vi "OCR Example.vi"() -> ()   [LabVIEW 2015]
doc: "This VI demonstrates how OCR could be used in an unstructured environment. Given the shape of surface that the text is printed on, LabVIEW can perform a perspective distortion correction to allow the OCR to better translate the text."
uses:
  <vilib>/userdefined/High Color/IMAQdx.ctl
  <vilib>/vision/driver/NI_Vision_Acquisition_Software.lvlib
  <resource>/objmgr/imaqdx.rc
  <vilib>/vision/NI_Vision_Development_Module.lvlib
panel:
  in  "stop":bool
  in  "Error in (no error)":errorcluster
  in  "Video Source":enum32{"File", "Live"}(radio)
  out "Camera Tab Control":enum32{"Pre-Loaded Video", "Live Camera"}(tab)
  in  "Frame Number":u32(slide) max=8 scale=0.0..8.0
  in  "Live Camera":T1="Select camera"
  in  "Video modes":u16(ring) items=["160x120 MJPG 30.00fps", "160x120 YUY2 30.00fps", "176x144 MJPG 30.00fps", "176x144 YUY2 30.00fps", "320x176 MJPG 30.00fps", "320x176 YUY2 30.00fps", "320x240 MJPG 30.00fps", "320x240 YUY2 30.00fps", "352x288 MJPG 30.00fps", "352x288 YUY2 30.00fps", "432x240 MJPG 30.00fps", "432x240 YUY2 30.00fps", "544x288 MJPG 30.00fps", "544x288 YUY2 30.00fps", "640x360 MJPG 30.00fps", "640x360 YUY2 30.00fps", "640x480 MJPG 30.00fps", "640x480 YUY2 30.00fps", "800x480 MJPG 30.00fps", "1024x768 MJPG 30.00fps"]
  in  "Start":bool
  in  "Tab Control":enum32{"Thresholding", "Corrected Feed"}(tab)=enum."Corrected Feed"
  out "Thresholded Image":T2(plugin-control)
  in  "Red or Hue":cluster{"Min":i32, "Max":i32}(slide)={"Min"=217, "Max"=15} scale=0.0..255.0
  in  "Green or Saturation":cluster{"Min":i32, "Max":i32}(slide)={"Min"=49, "Max"=165} scale=0.0..255.0
  in  "Blue or Luminance":cluster{"Min":i32, "Max":i32}(slide)={"Min"=65, "Max"=183} scale=0.0..255.0
  out "Corrected Feed":T2(plugin-control)
  in  "Relative Border Thickness":dbl(slide)=0.1274336283185841 scale=0.0..0.4 scale format="%.2g"
  out "OCR String":string
  out "Loop Time":i64
  in  "Apply correction":bool
  out "Original Feed":T2(plugin-control)
  # "This VI demonstrates how OCR could be used in an unstructured environment.\n  \n1. Select the video source before running the VI.\n2. Go through each frame without Apply correction toggled and notice when \nthe text is correctly identified.  \n3. Switch the image correction on.  Notice the change in Loop Time.\n\nThe video source must be live if using this example on an RT target.\nSee OCR Readme.html for more help and information."
  # "Use these sliders to adjust what color the \nVI identifies as the rectangle surrounding \nthe text."
  # "If using a Live video source, adjust the \nRelative Border Thickness so the green ROI\nlies completely within the red rectangle."
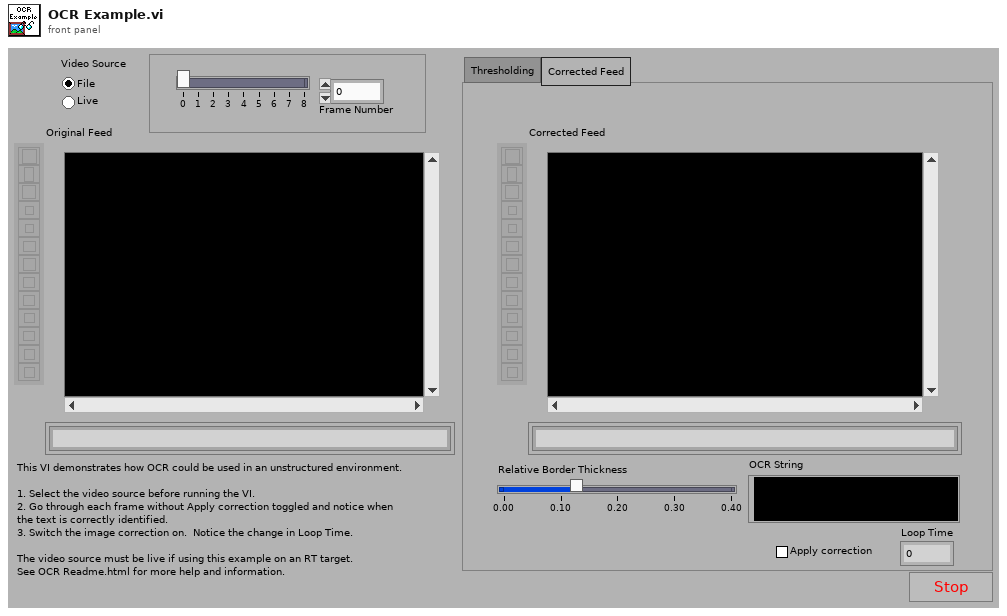
[diagram p1: front panel]
types:
  T1 = typedef "IMAQdx.ctl" = refnum<k21>
  T2 = typedef "IMAQ Image.ctl" = refnum<image>
  T3 = typedef "AviRefnum.ctl" = refnum<k1>
  T4 = typedef "IMAQ OCR Session.ctl" = refnum<k1>
  T5 = typedef "Image Type" = u32
  T6 = typedef "ROI Descriptor" = cluster{"Global Rectangle":i32[], "Contours":cluster{"ID":enum32{"External", "Internal"}, "Type":u32, "Coordinates":i32[]}[]}
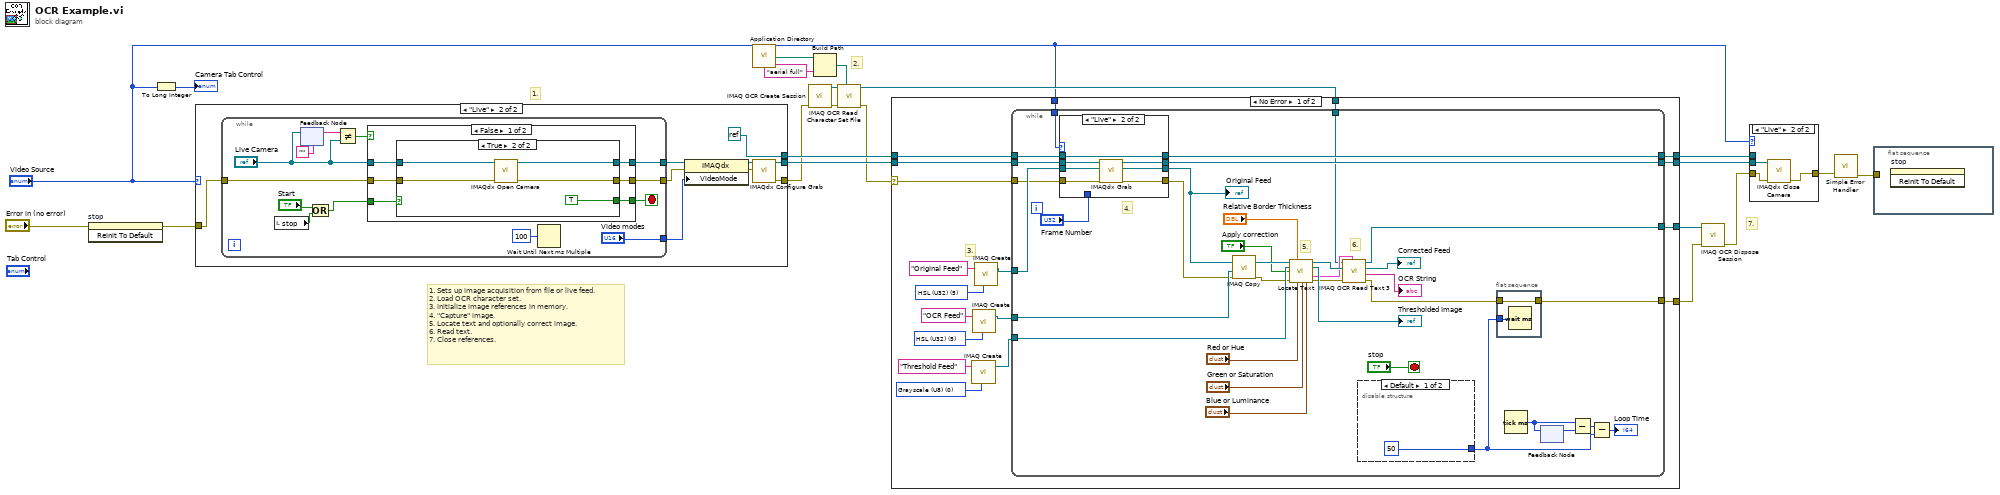
[diagram p0: block diagram]
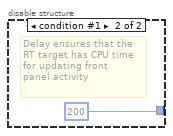
[diagram p2: hidden frame]
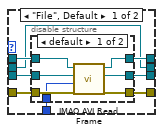
[diagram p3: hidden frame]
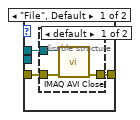
[diagram p6: hidden frame]
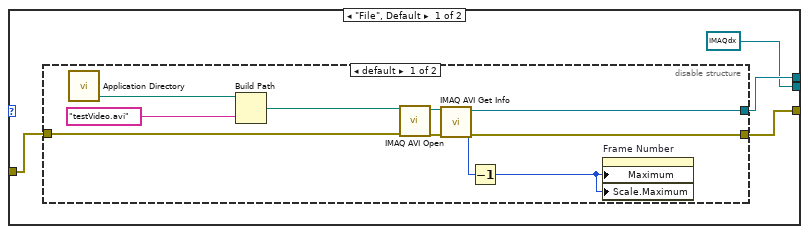
[diagram p8: hidden frame]
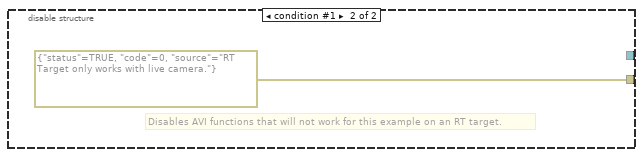
[diagram p9: hidden frame]
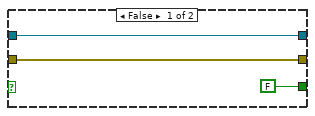
[diagram p10: hidden frame]
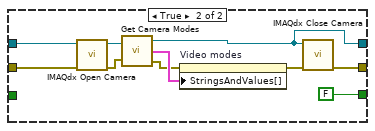
[diagram p11: hidden frame]
diagram:
  # "7."
  # "2."
  # "1."
  # "1. Sets up image acquisition from file or live feed.\n2. Load OCR character set.\n3. Initialize image references in memory.\n4. \"Capture\" image.\n5. Locate text and optionally correct image.\n6. Read text.\n7. Close references."
  n1 = invoke on="stop" class="Bool (strict)" method="Reinit To Default"(error in="Error in (no error)") -> (error out=w2:errorcluster)  [unwired: 2 in, 2 out]
  n2 = To Long Integer(number="Video Source") -> (32bit integer=→"Camera Tab Control":i32)
  n3 = case shown="\"Live\"" "Video Source" {
    tunnel: [T1 refnum ("Session Out") w45] -> w21
    tunnel: [w24 w42] -> w7
    tunnel: [w25 refnum<k0> refnum] -> w19
    tunnel: w2 -> [w23 w38]
    frame "File", Default {
      n4 = disable-structure shown="default" {
        disable-tunnel: [w34 _] -> w25
        disable-tunnel: [w33 errorcluster {"status"=TRUE, "code"=0, "source"="RT Target only works with live camera."} ("error out")] -> w24
        disable-tunnel: w23 -> [w26 _]
        frame condition #0 (active) {
          n5 = call <vilib>:"Application Directory.vi"() -> ("Application Directory"=w29:path)
          n6 = Build Path(base path=w29, name or relative path="testVideo.avi") -> (appended path=w27:path)
          n7 = call "IMAQ AVI Open"("error in (no error)"=w26, "AVI Path"=w27) -> ("error out"=w32:errorcluster, "Avi Refnum"=w35:T3)  [unwired: 8 in]
          n8 = call "IMAQ AVI Get Info"("error in (no error)"=w32, "Avi Refnum"=w35) -> ("error out"=w33:errorcluster, "Number of Frames"=w31:u32, "Avi Refnum (duplicate)"=w34:T3)  [unwired: 5 in, 2 out]
          n9 = Decrement(x=w31) -> (x-1=w30:u32)
          n10 = property on="Frame Number" class="Slide (strict)"("Maximum"=w30, "Scale.Maximum"=w30) -> ()  [unwired: 2 in, 2 out]
        }
        frame condition #1 {
          # "Disables AVI functions that will not work for this example on an RT target."
        }
      }
    }
    frame "Live" {
      n11 = while {
        tunnel: ["Video modes"] -> w41
        tunnel: [w52] -> w39
        tunnel: w38 -> [w54]
        tunnel: [w53] -> w40
        stop <- w50 stop-if-true
        n12 = local read "stop"() -> (w49:bool)
        n13 = feedback-in #1("Live Camera") -> ()
        n14 = feedback #1("") -> (w57:string)
        n15 = Or(x="Start", y=w49) -> (x .or. y?=w47:bool)
        n16 = Not Equal?(x=w57, y="Live Camera") -> (x != y?=w55:bool)
        n17 = case shown="False" w55 {
          tunnel: w54 -> [w61 w77]
          tunnel: [w60 w76] -> w53
          tunnel: [w62 w75] -> w52
          tunnel: "Live Camera" -> [w63 w74]
          tunnel: [w59 FALSE ("Start")] -> w50
          tunnel: w47 -> [w64 _]
          frame False {
            n18 = case shown="True" w64 {
              tunnel: w63 -> [w67 w72]
              tunnel: [w67 w71] -> w62
              tunnel: w61 -> [w66 w70]
              tunnel: [w66 w69] -> w60
              tunnel: [FALSE ("Start") TRUE ("Start")] -> w59
              frame False {
              }
              frame True {
                n19 = call <vilib>:"IMAQdx Open Camera.vi"("error in"=w70, "Session In"=w72) -> ("error out"=w69:errorcluster, "Session Out"=w71:T1)  [unwired: 8 in]
              }
            }
          }
          frame True {
            n20 = call <vilib>:"IMAQdx Open Camera.vi"("error in"=w77, "Session In"=w74) -> ("error out"=w80:errorcluster, "Session Out"=w81:T1)  [unwired: 8 in]
            n21 = call "Get Camera Modes.vi"("Session in"=w81, "Error in (no error)"=w80) -> ("Session Out"=w75:T1, "Video Modes out"=w79:cluster{"String":string, "Value":ext}[], "error out"=w78:errorcluster)
            n22 = property on="Video modes" class="Ring (strict)"(error in=w78, "StringsAndValues[]"=w79) -> (error out=w82:errorcluster)  [unwired: 1 in, 1 out]
            n23 = call <vilib>:"IMAQdx Close Camera.vi"("error in"=w82, "Session In"=w75) -> ("error out"=w76:errorcluster)  [unwired: 9 in]
          }
        }
        n24 = Wait Until Next ms Multiple(millisecond multiple=u32 100) -> ()  [unwired: 1 out]
      }
      n25 = property class="IMAQdx"(reference=w39, error in=w40, "VideoMode"=w41) -> (reference out=w44:T1, error out=w43:errorcluster)
      n26 = call <vilib>:"IMAQdx Configure Grab.vi"("error in"=w43, "Session In"=w44) -> ("error out"=w42:errorcluster, "Session Out"=w45:T1)  [unwired: 8 in]
    }
  }
  n27 = call <vilib>:"Application Directory.vi"() -> ("Application Directory"=w16:path)
  n28 = call "IMAQ OCR Create Session"("error in (no error)"=w7) -> ("error out"=w14:errorcluster, "IMAQ OCR Session"=w12:T4)  [unwired: 9 in]
  n29 = Build Path(base path=w16, name or relative path="aerial full") -> (appended path=w13:path)
  n30 = call "IMAQ OCR Read Character Set File"("File Path"=w13, "error in (no error)"=w14, "IMAQ OCR Session"=w12) -> ("error out"=w8:errorcluster, "IMAQ OCR Session (dup)"=w11:T4)  [unwired: 6 in, 1 out]
  n31 = case shown="No Error" w8 {
    selector: w8 -> [w93 w165]
    tunnel: w21 -> [w100 w166]
    tunnel: [w99 w166] -> w20
    tunnel: w19 -> [w98 w167]
    tunnel: [w97 w167] -> w18
    tunnel: w11 -> [w96 w168]
    tunnel: [w95 w168] -> w9
    tunnel: "Video Source" -> [w94 _]
    tunnel: [w92 w165] -> w6
    frame No Error {
      w90 = T5 5 items=["Grayscale (U8)", "Grayscale (I16)", "Grayscale (SGL)", "Complex (CSG)", "RGB (U32)", "HSL (U32)", "RGB (U64)", "Grayscale (U16)"] ("Image Type")
      w88 = T5 0 items=["Grayscale (U8)", "Grayscale (I16)", "Grayscale (SGL)", "Complex (CSG)", "RGB (U32)", "HSL (U32)", "RGB (U64)", "Grayscale (U16)"] ("Image Type")
      w87 = T5 5 items=["Grayscale (U8)", "Grayscale (I16)", "Grayscale (SGL)", "Complex (CSG)", "RGB (U32)", "HSL (U32)", "RGB (U64)", "Grayscale (U16)"] ("Image Type")
      # "3."
      n32 = call "IMAQ Create"("Image Name"="Threshold Feed", "Image Type"=w88) -> ("New Image"=w83:T2)  [unwired: 3 in, 1 out]
      n33 = call "IMAQ Create"("Image Name"="OCR Feed", "Image Type"=w90) -> ("New Image"=w84:T2)  [unwired: 3 in, 1 out]
      n34 = call "IMAQ Create"("Image Name"="Original Feed", "Image Type"=w87) -> ("New Image"=w85:T2)  [unwired: 3 in, 1 out]
      n35 = while {
        tunnel: w100 -> [w135]
        tunnel: [w134] -> w99
        tunnel: w85 -> [w133]
        tunnel: w83 -> [w132]
        tunnel: w84 -> [w131]
        tunnel: w93 -> [w130]
        tunnel: [w106] -> w92
        tunnel: w98 -> [w118]
        tunnel: [w117] -> w97
        tunnel: w94 -> [w115]
        tunnel: w96 -> [w109]
        tunnel: [w108] -> w95
        stop <- "stop" stop-if-true
        # "6."
        # "5."
        # "4."
        n36 = case shown="\"Live\"" w115 {
          tunnel: w135 -> [w140 w164]
          tunnel: [w140 w163] -> w134
          tunnel: w133 -> [w143 w162]
          tunnel: w130 -> [w147 w161]
          tunnel: [w145 w160] -> w129
          tunnel: [w146 w159] -> w127
          tunnel: w118 -> [w144 w158]
          tunnel: [w142 w158] -> w117
          tunnel: "Frame Number" -> [w141 _]
          frame "File", Default {
            n37 = disable-structure shown="default" {
              disable-tunnel: w147 -> [w154 w157]
              disable-tunnel: [w153 w157] -> w146
              disable-tunnel: [w152 w156] -> w145
              disable-tunnel: w144 -> [w151 w155]
              disable-tunnel: w143 -> [w150 w156]
              disable-tunnel: [w149 w155] -> w142
              disable-tunnel: w141 -> [w148 _]
              frame condition #0 (active) {
                n38 = call "IMAQ AVI Read Frame"("error in (no error)"=w154, "Frame Number"=w148, "Image"=w150, "Avi Refnum"=w151) -> ("error out"=w153:errorcluster, "Image Out"=w152:T2, "Avi Refnum (duplicate)"=w149:T3)  [unwired: 4 in, 1 out]
              }
              frame condition #1 {
              }
            }
          }
          frame "Live" {
            n39 = call <vilib>:"IMAQdx Grab.vi"("error in"=w161, "Image In"=w162, "Session In"=w164) -> ("error out"=w159:errorcluster, "Image Out"=w160:T2, "Session Out"=w163:T1)  [unwired: 5 in, 1 out]
          }
        }
        "Original Feed" <- w129
        n40 = call "IMAQ Copy"("error in (no error)"=w127, "Image Dst"=w131, "Image Src"=w129) -> ("error out"=w126:errorcluster, "Image Dst Out"=w128:T2)  [unwired: 3 in]
        n41 = call "Locate Text.vi"("OCR Image"=w128, "Relative Border Thickness"="Relative Border Thickness", "Threshold image"=w132, "Correct Image?"="Apply correction", "error in (no error)"=w126, "Red or Hue"="Red or Hue", "Green or Saturation"="Green or Saturation", "Blue or Luminance"="Blue or Luminance") -> ("Corrected image"=w114:T2, "Threshed Image"=→"Thresholded Image":T2, "ROI Descriptor"=w110:T6, "error out"=w111:errorcluster)  [unwired: 4 in]
        n42 = call "IMAQ OCR Read Text 3"("ROI Descriptor"=w110, "error in (no error)"=w111, "Image"=w114, "IMAQ OCR Session"=w109) -> ("error out"=w107:errorcluster, "Read String"=→"OCR String":string, "Image (dup)"=→"Corrected Feed":T2, "IMAQ OCR Session (dup)"=w108:T4)  [unwired: 2 in, 2 out]
        n43 = disable-structure shown="Default" {
          disable-tunnel: [u32 50 ("milliseconds to wait") u32 200 ("milliseconds to wait")] -> w102
          frame condition #0 (active) {
          }
          frame condition #1 {
            # "Delay ensures that the\nRT target has CPU time\nfor updating front\npanel activity"
          }
        }
        n44 = flat-sequence {
          tunnel: w107 -> [w137]
          tunnel: [w137] -> w106
          tunnel: w102 -> [w136]
          frame #0 {
            n45 = Wait (ms)(milliseconds to wait=w136) -> ()  [unwired: 1 out]
          }
        }
        n46 = Tick Count (ms)() -> (millisecond timer value=w105:u32)
        n47 = feedback-in #2(w105) -> ()
        n48 = feedback #2() -> (w104:u32)  [unwired: 1 in]
        n49 = Subtract(x=w105, y=w104) -> (x-y=w103:u32)
        n50 = Subtract(x=w103, y=w102) -> (x-y=→"Loop Time":u32)
      }
    }
    frame Error {
    }
  }
  n51 = call "IMAQ OCR Dispose Session"("error in (no error)"=w6, "IMAQ OCR Session"=w9) -> ("error out"=w10:errorcluster)  [unwired: 9 in]
  n52 = case shown="\"Live\"" "Video Source" {
    tunnel: w20 -> [_ w178]
    tunnel: w10 -> [w171 w177]
    tunnel: w18 -> [w170 _]
    tunnel: [w169 w176] -> w15
    frame "File", Default {
      n53 = disable-structure shown="default" {
        disable-tunnel: w171 -> [w174 w175]
        disable-tunnel: w170 -> [w173 _]
        disable-tunnel: [w172 w175] -> w169
        frame condition #0 (active) {
          n54 = call "IMAQ AVI Close"("error in (no error)"=w174, "Avi Refnum"=w173) -> ("error out"=w172:errorcluster)  [unwired: 9 in]
        }
        frame condition #1 {
        }
      }
    }
    frame "Live" {
      n55 = call <vilib>:"IMAQdx Close Camera.vi"("error in"=w177, "Session In"=w178) -> ("error out"=w176:errorcluster)  [unwired: 9 in]
    }
  }
  n56 = call <vilib>:"Simple Error Handler.vi"("error in (no error)"=w15) -> ("error out"=w1:errorcluster)  [unwired: 4 in, 4 out]
  n57 = flat-sequence {
    tunnel: w1 -> [_]
    frame #0 {
      n58 = invoke on="stop" class="Bool (strict)" method="Reinit To Default"() -> ()  [unwired: 3 in, 3 out]
    }
  }
